vi "Get Axis Properties.vi"(8 "error in (no error)":errorcluster, 11 "Scale Refnum":refnum<vi>) -> (0 "error out":errorcluster, 3 "Axis Properties":T1)   [LabVIEW 2020]
uses:
  Axis Properties.ctl
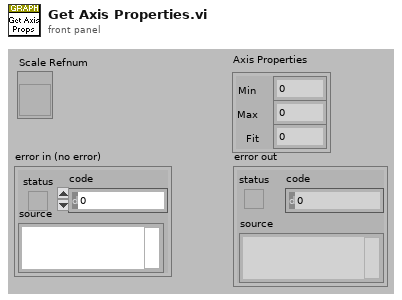
[diagram p1: front panel]
types:
  T1 = typedef "Axis Properties.ctl" = cluster{"Min":dbl, "Max":dbl, "Fit":u8}
  T2 = cluster{"Minimum":dbl, "Maximum":dbl, "ScaleFit":u8}
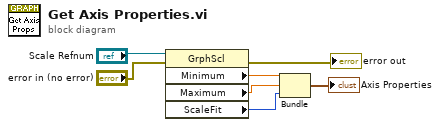
[diagram p0: block diagram]
diagram:
  n1 = property class="GrphScl"(reference="Scale Refnum", error in="error in (no error)") -> (error out=→"error out":errorcluster, "Minimum"=w5:dbl, "Maximum"=w4:dbl, "ScaleFit"=w3:u8)  [unwired: 1 out]
  n2 = Bundle("Minimum"=w5, "Maximum"=w4, "ScaleFit"=w3) -> (→"Axis Properties":T2)  [unwired: 1 in]
